vi "Dark Current Test (Brute Force Version).vi"() -> ()   [LabVIEW 2020]
uses:
  <vilib>/DAQmx/create/channels.llb/DAQmx Create Channel (DO-Digital Output).vi
panel:
  out "Individual Tube \nCurrent (Nano Amps)":dbl[](array[numeric])
  out "Test Is Running (Red)\nTest Is Stopped (Green)":bool
  in  "Start":bool
  out "Failed Tubes":string[](array[string])
  in  "Barcodes in 4":string[](array[string])
  in  "Barcodes in 3":string[](array[string])
  in  "Barcodes in 2":string[](array[string])
  in  "Barcodes in":string[](array[string])
  out "Actual Voltage Level (V)":dbl format="%#_13g"
  out "Power Supply Trip":bool
  out "Actual Current Limit (nA)":dbl format="%#_13g"
  out "Mesurnment Iteration":i32
  in  "stop":bool
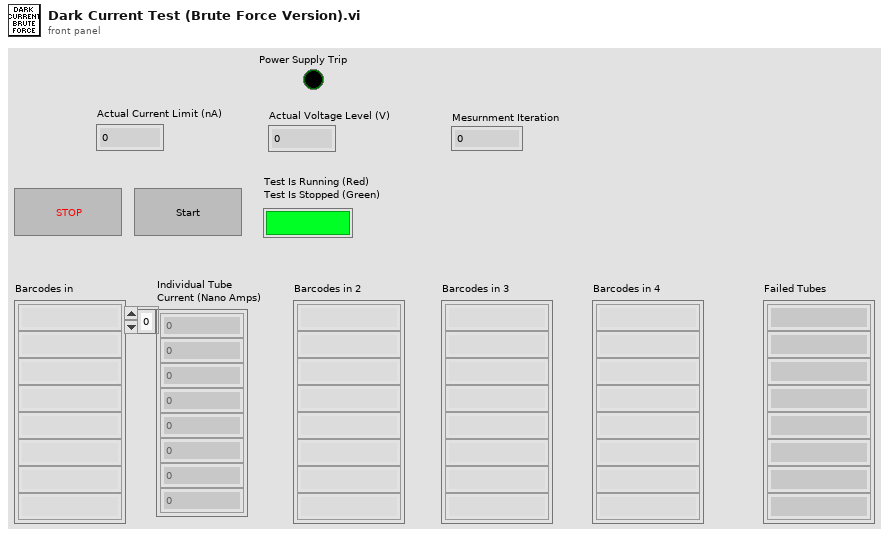
[diagram p1: front panel]
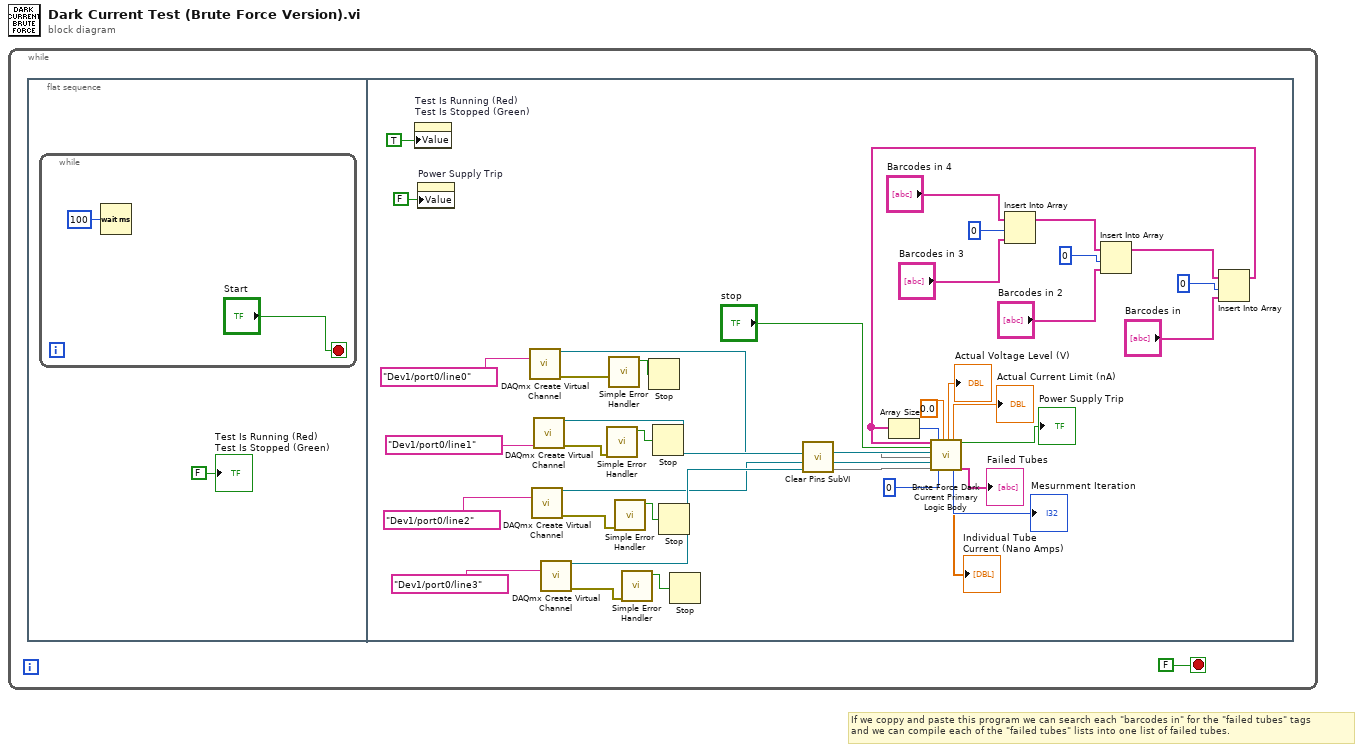
[diagram p0: block diagram]
diagram:
  # "If we coppy and paste this program we can search each \"barcodes in\" for the \"failed tubes\" tags\nand we can compile each of the \"failed tubes\" lists into one list of failed tubes."
  n1 = while {
    stop <- FALSE stop-if-true
    n2 = flat-sequence {
      frame #0 {
        n3 = while {
          stop <- "Start" stop-if-true
          n4 = Wait (ms)(milliseconds to wait=u32 100) -> ()  [unwired: 1 out]
        }
        "Test Is Running (Red)\nTest Is Stopped (Green)" <- FALSE ("Start LED")
      }
      frame #1 {
        n5 = property on="Test Is Running (Red)\nTest Is Stopped (Green)" class="Bool (strict)"("Value"=TRUE) -> ()  [unwired: 2 in, 2 out]
        n6 = property on="Power Supply Trip" class="Bool (strict)"("Value"=FALSE ("Power Supply Trip")) -> ()  [unwired: 2 in, 2 out]
        n7 = call-poly <vilib>:"DAQmx Create Virtual Channel.vi"("lines"=tag "Dev1/port0/line0" ("Data Pin")) -> ("task out"=w20:refnum<k21>, "error out"=w40:errorcluster)  [unwired: 13 in]
        n8 = call-poly <vilib>:"DAQmx Create Virtual Channel.vi"("lines"=tag "Dev1/port0/line2" ("Write Pin")) -> ("task out"=w18:refnum<k21>, "error out"=w38:errorcluster)  [unwired: 13 in]
        n9 = call-poly <vilib>:"DAQmx Create Virtual Channel.vi"("lines"=tag "Dev1/port0/line1" ("Sync Pin")) -> ("task out"=w32:refnum<k21>, "error out"=w39:errorcluster)  [unwired: 13 in]
        n10 = call-poly <vilib>:"DAQmx Create Virtual Channel.vi"("lines"=tag "Dev1/port0/line3" ("Clear Pin")) -> ("task out"=w31:refnum<k21>, "error out"=w37:errorcluster)  [unwired: 13 in]
        n11 = call <vilib>:"Simple Error Handler.vi"("error in (no error)"=w39) -> ("error?"=w33:bool)  [unwired: 4 in, 4 out]
        n12 = call <vilib>:"Simple Error Handler.vi"("error in (no error)"=w40) -> ("error?"=w36:bool)  [unwired: 4 in, 4 out]
        n13 = call <vilib>:"Simple Error Handler.vi"("error in (no error)"=w38) -> ("error?"=w34:bool)  [unwired: 4 in, 4 out]
        n14 = call <vilib>:"Simple Error Handler.vi"("error in (no error)"=w37) -> ("error?"=w35:bool)  [unwired: 4 in, 4 out]
        n15 = Stop(stop? (T)=w36) -> ()
        n16 = Stop(stop? (T)=w33) -> ()
        n17 = Stop(stop? (T)=w34) -> ()
        n18 = Stop(stop? (T)=w35) -> ()
        n19 = call "Clear Pins SubVI.vi"(8:w31, 10:w32) -> (0:w17, 2:w19)  [unwired: 7 in, 1 out]
        n20 = Insert Into Array(array="Barcodes in 4", index=0, new element="Barcodes in 3") -> (w26:string[])
        n21 = Insert Into Array(array=w26, index=0, new element="Barcodes in 2") -> (w22:string[])
        n22 = Insert Into Array(array=w22, index=0, new element="Barcodes in") -> (w16:string[])
        n23 = Array Size(array=w16) -> (size(s)=w14:i32)
        n24 = call "Brute Force Dark Current Primary Logic Body.vi"("Barcodes in"=w16, "stop"="stop", "Pins In"=w20, 3:w19, 4:w18, "VISA Refnum in"=w17, "Number of Tubes"=w14, "Channel #"=0, 8:0.0 ("Trip Count")) -> ("Actual Voltage Level (V)"=→"Actual Voltage Level (V)":dbl, "Individual Tube Current (Nano Amps)"=→"Individual Tube \nCurrent (Nano Amps)":dbl[], "Actual Current Limit (nA)"=→"Actual Current Limit (nA)":dbl, "Mesurnment Iteration"=→"Mesurnment Iteration":i32, "Power Supply Trip"=→"Power Supply Trip":bool, "Failed Tubes"=→"Failed Tubes":string[])  [unwired: 4 in, 1 out]
      }
    }
  }
